vi "get FP controls.vi"(8 "error in (no error)":errorcluster, 11 "VI in":refnum<vi>) -> (0 "error out":errorcluster, 3 "Controls[]":refnum<vi>[](array[refnum]))   [LabVIEW 2013, in "NISE Tools Scripting.lvlib"]
uses:
  NISE Tools Scripting.lvlib
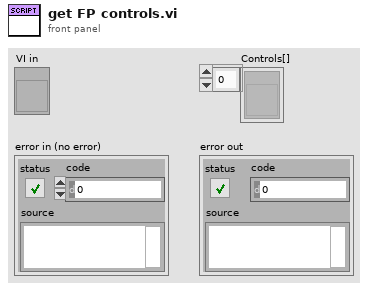
[diagram p1: front panel]
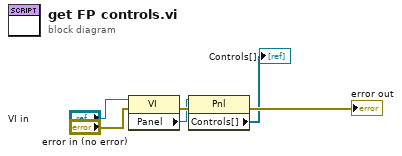
[diagram p0: block diagram]
diagram:
  n1 = property class="VI"(reference="VI in", error in="error in (no error)") -> (error out=w5:errorcluster, "Panel"=w1:refnum<vi>)  [unwired: 1 out]
  n2 = property class="Pnl"(reference=w1, error in=w5) -> (error out=→"error out":errorcluster, "Controls[]"=→"Controls[]":refnum<vi>[])  [unwired: 1 out]
